vi "1SDI_Output_v00.vi"(8 "Outputs":T2, 11 "Safety First":T1) -> ()   [LabVIEW 2013]
doc: "Outputs the signals to FPGA output nodes, after a variable rate-limiter has been applied."
uses:
  Strict Type Defs/1SDI Output.ctl
  Strict Type Defs/Safety First.ctl
  <vilib>/rvi/eio/common/nirviEmuTemplateMethod_errors.vi
  <vilib>/rvi/Analysis/common/FxpNativeNode/niFpgaFxpNative.xnode
  <vilib>/eio/EIONode/EIONode.xnode
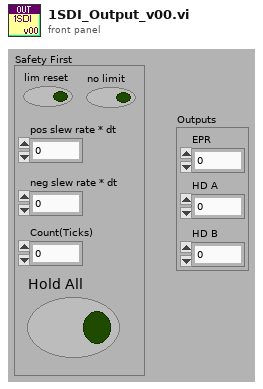
[diagram p1: front panel]
types:
  T1 = typedef "Safety First.ctl" = cluster{"lim reset":bool, "no limit":bool, "pos slew rate * dt":i16, "neg slew rate * dt":i16, "Hold All":bool, "Count(Ticks)":u32}
  T2 = typedef "1SDI Output.ctl" = cluster{"EPR":i16, "HD A":i16, "HD B":i16}
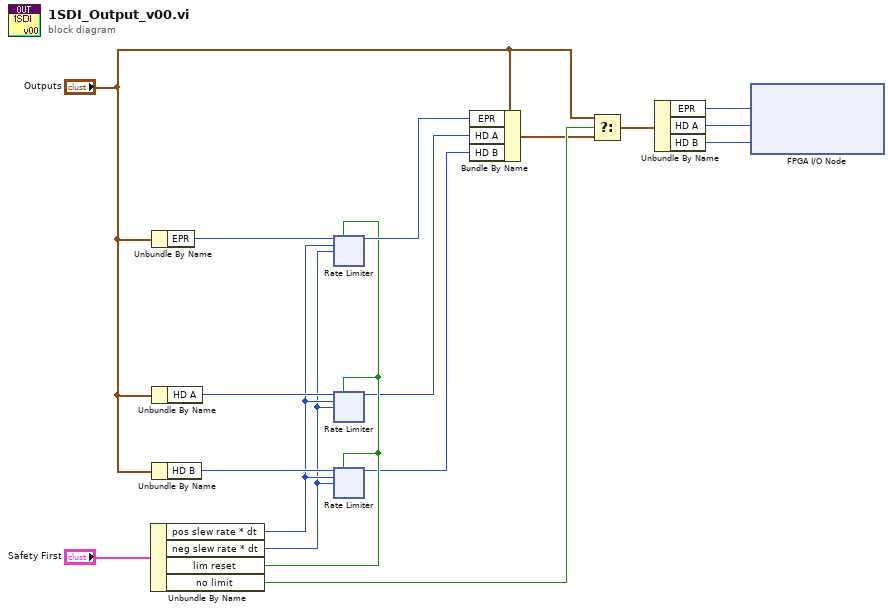
[diagram p0: block diagram]
diagram:
  n1 = Unbundle By Name("Safety First") -> ("pos slew rate * dt"=w4:i16, "neg slew rate * dt"=w3:i16, "lim reset"=w5:bool, "no limit"=w14:bool)
  n2 = Unbundle By Name("Outputs") -> ("EPR"=w16:i16)
  n3 = Unbundle By Name("Outputs") -> ("HD A"=w7:i16)
  n4 = Unbundle By Name("Outputs") -> ("HD B"=w8:i16)
  n5 = xnode ("Rate Limiter")("pos slew rate * dt"=w4, "input"=w16, "neg slew rate * dt"=w3, "reset"=w5) -> ("output"=w15:i16)
  n6 = xnode ("Rate Limiter")("pos slew rate * dt"=w4, "input"=w7, "neg slew rate * dt"=w3, "reset"=w5) -> ("output"=w2:i16)
  n7 = xnode ("Rate Limiter")("pos slew rate * dt"=w4, "input"=w8, "neg slew rate * dt"=w3, "reset"=w5) -> ("output"=w1:i16)
  n8 = Bundle By Name(cluster="Outputs", "EPR"=w15, "HD A"=w2, "HD B"=w1) -> (w9:T2)
  n9 = Select(t="Outputs", s=w14, f=w9) -> (s? t:f=w13:T2)
  n10 = Unbundle By Name(w13) -> ("EPR"=w12:i16, "HD A"=w11:i16, "HD B"=w10:i16)
  n11 = xnode "FPGA I/O Node"("Connector0/AO0"=w12, "Connector0/AO1"=w11, "Connector0/AO2"=w10) -> ()  [unwired: 3 in, 3 out]
